vi "Read Power.vi"(8 "error in (no error)":errorcluster, 11 "LaserPower in":refnum<class "LaserPower.lvclass">) -> (0 "error out":errorcluster, 2 "Power":u8 caption="Power [8bit]", 3 "LaserPower out":refnum<class "LaserPower.lvclass">)   [LabVIEW 2013, in "HardwareCharacterization.lvlib" / "LaserPower.lvclass"]
uses:
  LaserPower.lvclass
  LaserPower.lvclass/LaserPower.ctl
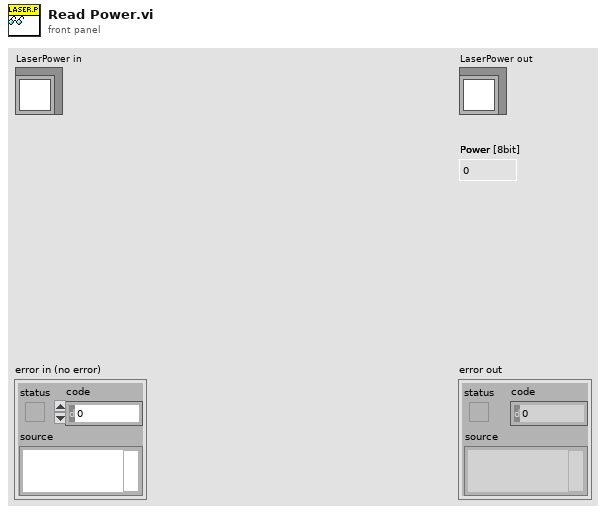
[diagram p1: front panel]
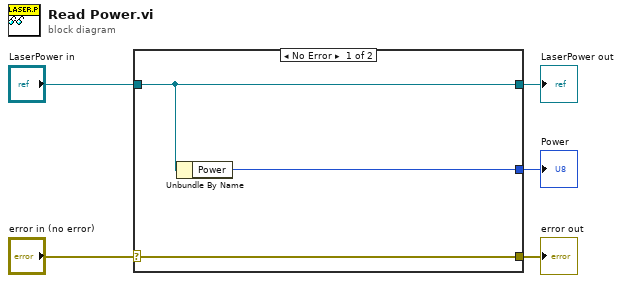
[diagram p0: block diagram]
diagram:
  n1 = case shown="No Error" "error in (no error)" {
    selector: "error in (no error)" -> [w8 w9]
    tunnel: [w8 w9] -> w4
    tunnel: [w7 w10] -> w2
    tunnel: "LaserPower in" -> [w7 w10]
    tunnel: [w6 _] -> w1
    frame No Error {
      n2 = Unbundle By Name(w7) -> ("Power"=w6:u8)
    }
    frame Error {
    }
  }
  "error out" <- w4
  "LaserPower out" <- w2
  "Power" <- w1
